vi "Visualizacion_NEW.vi"() -> ()   [LabVIEW 2022 SP3]
uses:
  4cb8985d-a683-42ab-be0b-9e8f42a2c2d0.vi
  <vilib>/Analysis/baseanly.llb/Mean (DBL).vi
  <vilib>/Modbus/master/Create Master Instance (TCP).vi
  <vilib>/Comparison/Less/Less Functor/Less Functor.lvclass
  <vilib>/Modbus/master/Modbus Master.lvclass
  <vilib>/Analysis/NI_AALBase.lvlib
panel:
  out "Temp V8":dbl(slide) scale=-40.0..100.0
  out "Temp BOB8":dbl(slide) scale=-40.0..100.0
  out "Temp BOB7":dbl(slide) scale=-40.0..100.0
  out "Temp V7":dbl(slide) scale=-40.0..100.0
  out "Temp V6":dbl(slide) scale=-40.0..100.0
  out "Temp BOB6":dbl(slide) scale=-40.0..100.0
  out "Temp BOB5":dbl(slide) scale=-40.0..100.0
  out "Temp V5":dbl(slide) scale=-40.0..100.0
  out "Temp BOB4":dbl(slide) scale=-40.0..100.0
  out "Temp V4":dbl(slide) scale=-40.0..100.0
  out "Temp V3":dbl(slide) scale=-40.0..100.0
  out "Temp BOB3":dbl(slide) scale=-40.0..100.0
  out "Temp BOB2":dbl(slide) scale=-40.0..100.0
  out "Temp V2":dbl(slide) scale=-40.0..100.0
  out "Temp V1":dbl(slide) scale=-40.0..100.0
  out "Temp BOB1":dbl(slide) scale=-40.0..100.0
  in  "Activar sim Bitron":bool
  out "MEDIA TEMPERATURAS":dbl format="%0.2f"
  out "Peltiers enable":bool
  out "Program Status":bool
  out "SP (T)":sgl
  out "Segmento_temp":u16
  in  "?":T1(tab)
  in  "?":T2(tab)
  out "TEMPERATURA MEDIA":dynamicdata(graph)
  out "ALL TOGETHER":dynamicdata(graph)
  out "VALVULA 1 Y BOBINA 1":dynamicdata(graph)
  out "VALVULA 2 Y BOBINA 2":dynamicdata(graph)
  out "VALVULA 3 Y BOBINA 3":dynamicdata(graph)
  out "VALVULA 4 Y BOBINA 4":dynamicdata(graph)
  out "VALVULA 5  Y BOBINA 5":dynamicdata(graph)
  out "VALVULA 6 Y BOBINA 6":dynamicdata(graph)
  out "VALVULA 7 Y BOBINA 7":dynamicdata(graph)
  out "VALVULA 8 Y PELTIER 8":dynamicdata(graph)
  out "Camara climatica":dynamicdata(graph)
  out "W1.16":bool
  out "W1.15":bool
  out "W1.11":bool
  out "1.10":bool
  out "W1.14":bool
  out "W1.13":bool
  out "W1.12":bool
  out "W1.1":bool
  out "W2":bool
  out "W3":bool
  out "W4":bool
  out "W1.2":bool
  out "W1.3":bool
  out "W1.6":bool
  out "W1.5":bool
  out "W1.4":bool
  out "W1.9":bool
  out "W1.8":bool
  out "W1.7":bool
  out "warnings table":T3(array[cluster]) {"Time Stamp" format="%<%.3X %x>T"}
  in  "Reset":bool
  in  "Pelt ºC/min":dbl=2.5
  in  "Cam ºC/min":dbl=2.2
  in  "Tiempo máximo de ciclo(min)":dbl=90.0
  in  "Setpoint corte frío(ºC)":dbl=-30.0
  in  "Setpoint Frío(ºC)":dbl=-40.0
  in  "Setpoint peltiers(ºC)":dbl=85.0
  in  "Tiempo estabilidad de Frío(min)":dbl=15.0
  in  "Tiempo mínimo de ciclo(min)":dbl=70.0
  in  "Setpoint calor corte rampa(ºC)":dbl=51.0
  in  "T ciclo (Bitron FSM Sim)":dbl=90.0
  in  "Setpoint calor cam":dbl=55.0
  in  "Save Parameters":bool
  out "DO H2 Lab":bool
  in  "?":T4(tab)
  out "Temp Valve 1":sgl format="%#.2g"
  out "Temp Bobina 1":sgl
  out "PWM 1(SP)":u16
  out "PWM 2(SP)":u16
  out "Temp Valve 2":sgl format="%#.2g"
  out "Temp Bobina 2":sgl
  out "PWM 3(SP)":u16
  out "Temp Valve 3":sgl format="%#.2g"
  out "Temp Bobina 3":sgl
  out "PWM 4(SP)":u16
  out "Temp Valve 4":sgl format="%#.2g"
  out "Temp Bobina 4":sgl
  out "Temp Valve 5":sgl
  out "Temp Bobina 5":sgl
  out "PWM 5(SP)":u16
  out "PWM 6(SP)":u16
  out "Temp Valve 6":sgl format="%#.2g"
  out "Temp Bobina 6":sgl
  out "PWM 7(SP)":u16
  out "Temp Valve 7":sgl format="%#.2g"
  out "Temp Bobina 7":sgl
  out "PWM 8(SP)":u16
  out "Temp Bobina 8":sgl
  out "Temp Valve 8":sgl format="%#.2g"
  in  "Guardar datos":bool=TRUE
  out "Array":dbl[][](array[numeric])
  out "Guardando en disco":bool
  out "array w/ subset deleted":dbl[][](array[numeric])
  out "Guardar Array":dbl[][](array[numeric])
  out "size(s)":i32
  out "senal_bitron":bool
  in  "Stop Control Program":bool
  out "Coils write":bool[](array[boolean])
  out "error out":errorcluster
  out "Int values":u16[](array[numeric])
  out "SGL values":sgl[](array[numeric])
  out "coil values":bool[](array[boolean])
  out "ComunicacionCRIO":bool
  out "current time":timestamp
  in  "run_program":bool
  out "Setpoint_temp_write":dbl
  out "Setpoint_hum_write":dbl
  out "Setpoint_temp_read":dbl
  out "Setpoint_hum_read":dbl
  in  "Pause_Entrar_camara":bool
  in  "Pause":bool
  in  "stop":bool
  # "Control Programa Principal"
  # "Cámara climática"
  # "ºC"
  # "ºC"
  # "%"
  # "%"
  # "Simulación señal Bitron"
  # "ºC"
  # "1            2          3           4           5          6          7          8"
  # "T Manifolds"
  # "1            2          3           4           5          6          7          8"
  # "T Bobinas"
  # "Warnings y Errores"
  # "Parametros y configuracion para la curva de ciclado"
  # "Peltier 1"
  # "ºC"
  # "ºC"
  # "Peltier 2"
  # "ºC"
  # "ºC"
  # "Peltier 3"
  # "ºC"
  # "ºC"
  # "Peltier 4"
  # "ºC"
  # "ºC"
  # "Peltier 5 (Doble)"
  # "ºC"
  # "ºC"
  # "Peltier 6 (Doble)"
  # "ºC"
  # "ºC"
  # "Peltier 7 (Doble)"
  # "ºC"
  # "ºC"
  # "Peltier 8 (Doble)"
  # "ºC"
  # "ºC"
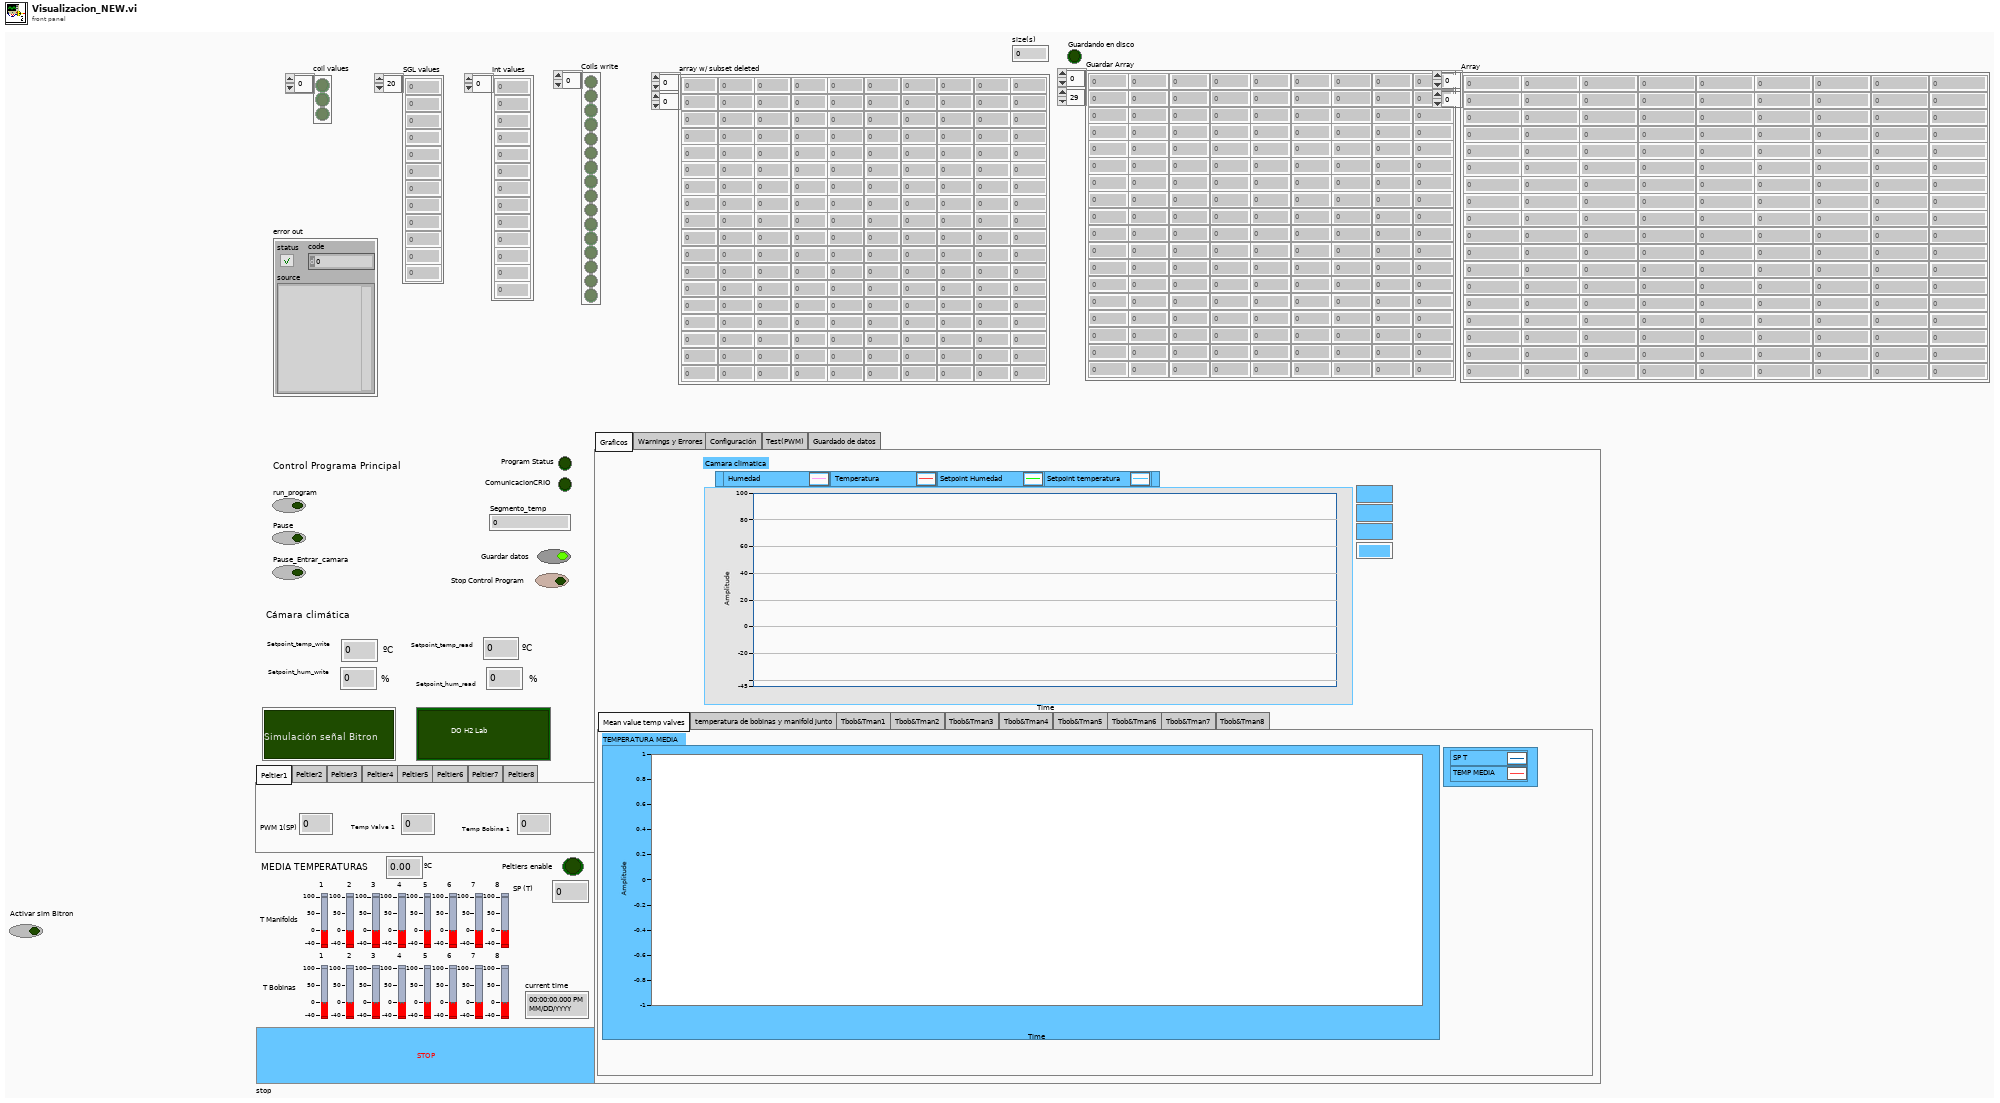
[diagram p1: front panel]
types:
  T1 = enum32{"Graficos", "Warnings y Errores", "Configuración", "Test(PWM)", "Guardado de datos"}
  T2 = enum32{"Mean value temp valves", "temperatura de bobinas y manifold junto", "Tbob&Tman1", "Tbob&Tman2", "Tbob&Tman3", "Tbob&Tman4", "Tbob&Tman5", "Tbob&Tman6", "Tbob&Tman7", "Tbob&Tman8"}
  T3 = cluster{"Time Stamp":timestamp, "Descripcion":string, "Numeric":i32}[]
  T4 = enum32{"Peltier1", "Peltier2", "Peltier3", "Peltier4", "Peltier5", "Peltier6", "Peltier7", "Peltier8"}
  T5 = enum16{"open", "open or create", "create or replace", "create", "open (read-only)"}
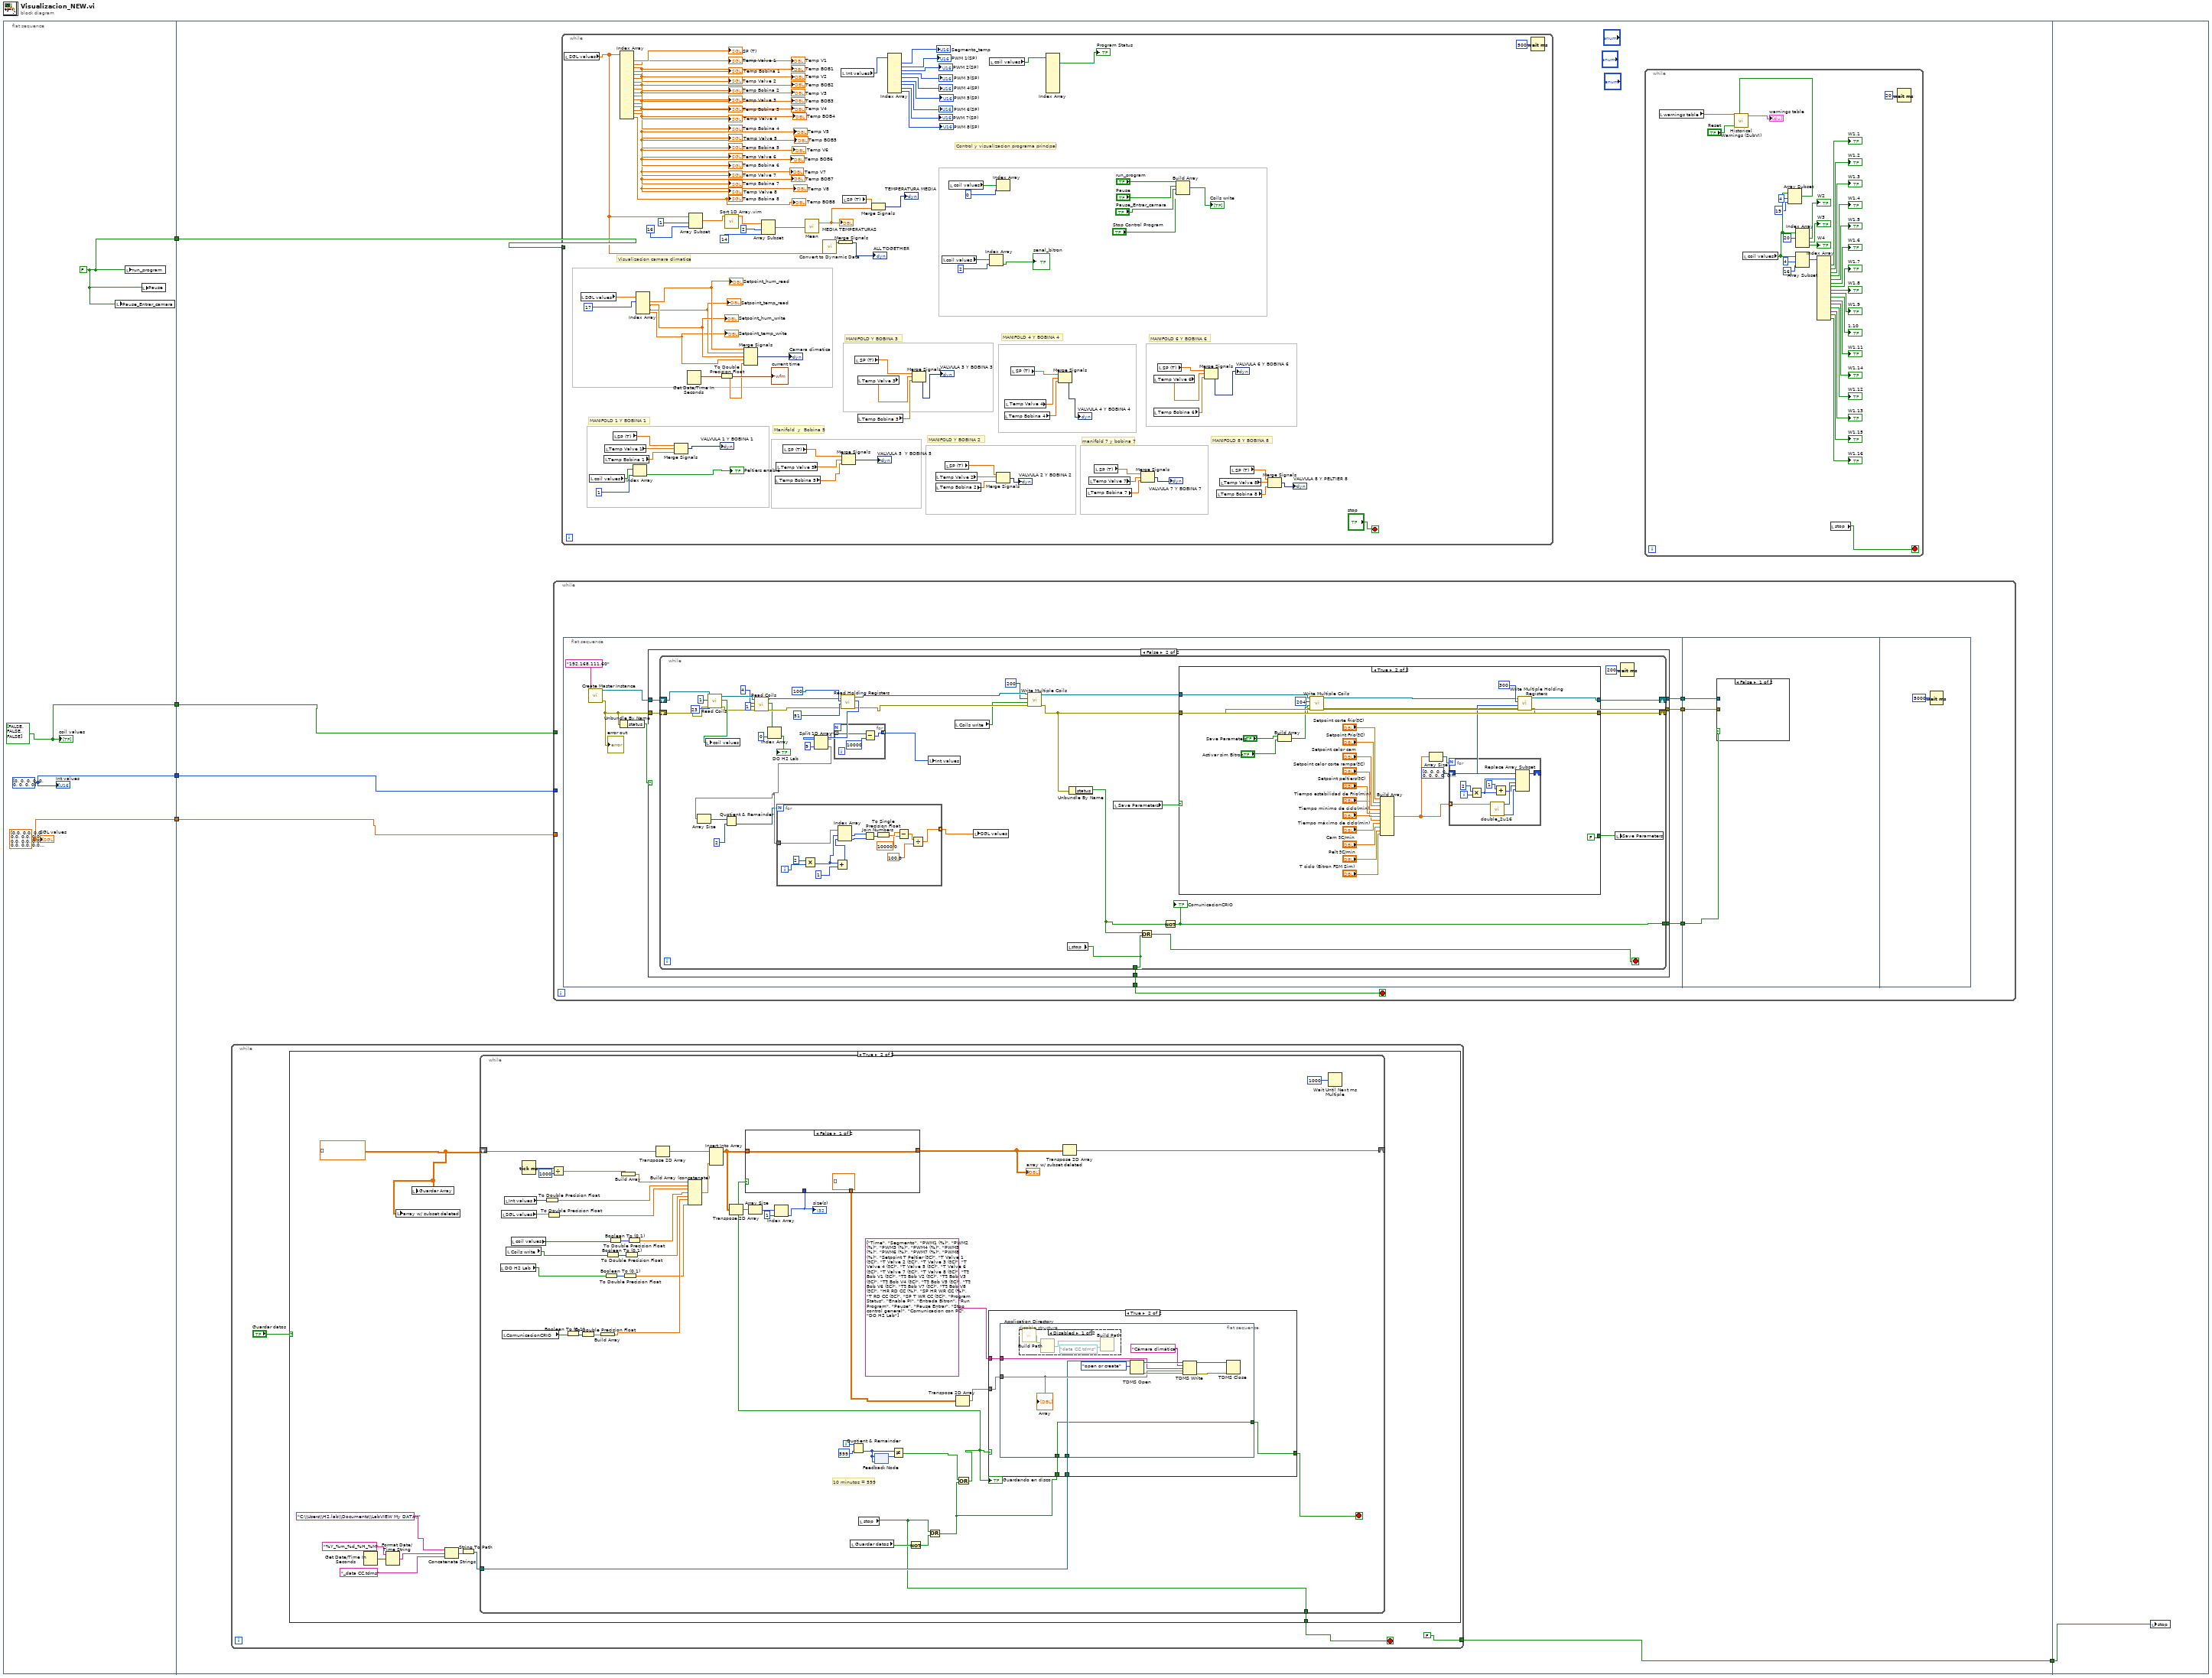
[diagram p0: block diagram]
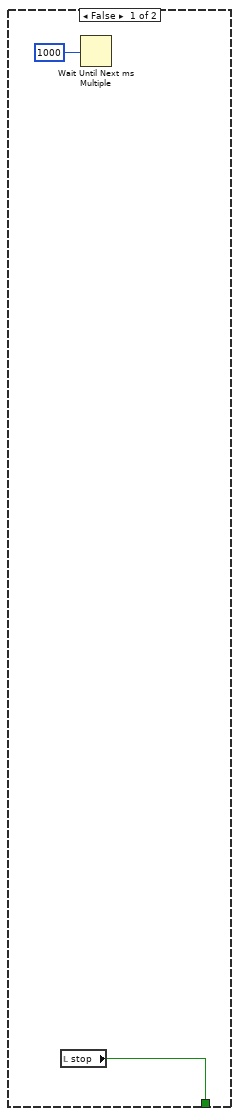
[diagram p2: hidden frame]
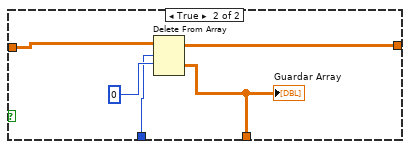
[diagram p3: hidden frame]
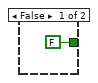
[diagram p4: hidden frame]
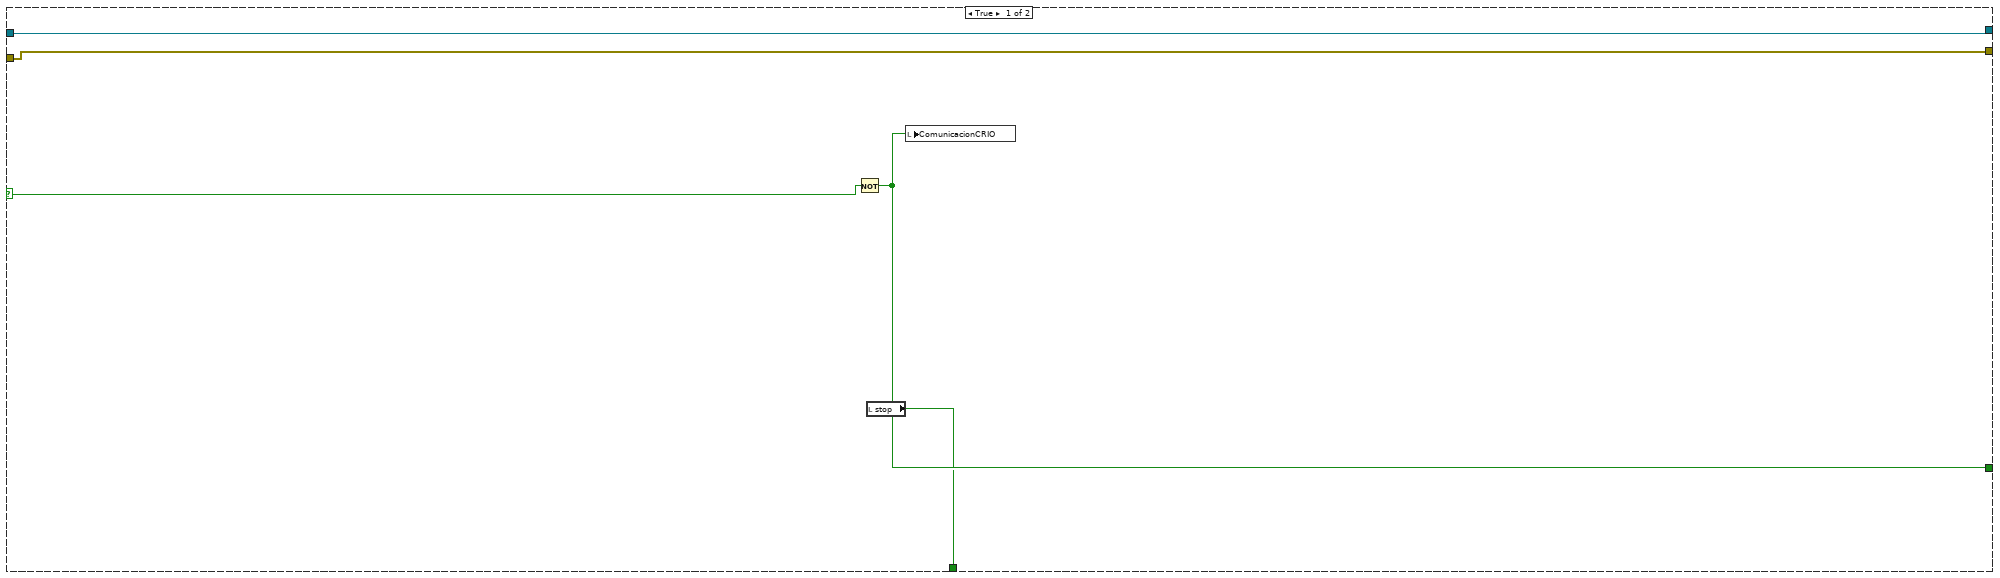
[diagram p6: hidden frame]
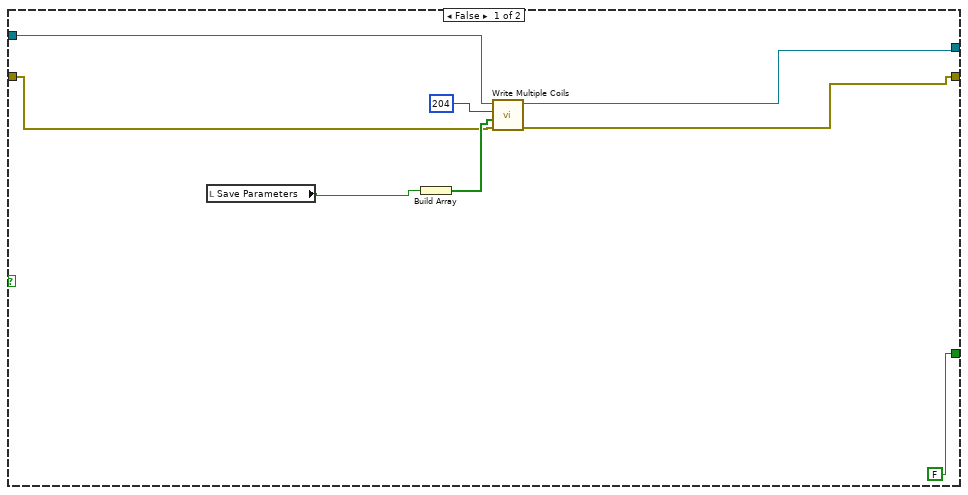
[diagram p7: hidden frame]
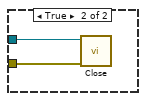
[diagram p8: hidden frame]
diagram:
  n1 = flat-sequence {
    tunnel: [w9] -> w5
    tunnel: [w8] -> w4
    tunnel: [w7] -> w3
    tunnel: [w6] -> w2
    tunnel: w5 -> [w14]
    tunnel: w4 -> [w13]
    tunnel: w3 -> [w12]
    tunnel: w2 -> [w11]
    tunnel: [w10] -> w1
    tunnel: w1 -> [w363]
    frame #0 {
      w7 = sgl[] [0.0, 0.0, 0.0, 0.0, 0.0, 0.0, 0.0, 0.0, 0.0, 0.0, 0.0, 0.0, 0.0, 0.0, 0.0, 0.0, 0.0, 0.0, 0.0, 0.0, 0.0] ("SGL values")
      w8 = u16[] [0, 0, 0, 0, 0, 0, 0, 0, 0] ("Int values")
      w6 = FALSE ("run_program")
      w9 = bool[] [FALSE, FALSE, FALSE] ("coil values")
      n2 = local write "Pause_Entrar_camara"(w6) -> ()
      n3 = local write "run_program"(w6) -> ()
      n4 = local write "Pause"(w6) -> ()
      "coil values" <- w9
      "Int values" <- w8
      "SGL values" <- w7
    }
    frame #1 {
      n5 = while {
        tunnel: [FALSE ("stop Control General")] -> w10
        stop <- w48 stop-if-true
        n6 = case shown="True" "Guardar datos" {
          tunnel: [w50 w52] -> w48
          frame False {
            n7 = local read "stop"() -> (w50:bool)
            n8 = Wait Until Next ms Multiple(millisecond multiple=u32 1000 ("milliseconds to wait")) -> ()  [unwired: 1 out]
          }
          frame True {
            w60 = dbl[][] []
            n9 = Get Date/Time In Seconds() -> (seconds since 1Jan1904=w59:timestamp)
            n10 = Format Date/Time String(time format string (%c)="%Y_%m_%d_%H_%M", seconds (now)=w59) -> (date/time string=w56:string)  [unwired: 1 in]
            n11 = local write "array w/ subset deleted"(w60) -> ()
            n12 = local write "Guardar Array"(w60) -> ()
            n13 = Concatenate Strings("C:\\Users\\H2.lab\\Documents\\LabVIEW My DATA\\" ("string"), w56, "_data CC.tdms" ("string")) -> (w57:string)
            n14 = String To Path(string=w57) -> (path=w54:path)
            n15 = while {
              shift-right: [w97] -> _
              shift-left: w60 -> [w100]
              tunnel: w54 -> [w88]
              tunnel: [w64] -> w52
              i -> [w105]
              stop <- w68 stop-if-true
              # "10 minutos = 599"
              n16 = local read "DO H2 Lab"() -> (w62:bool)
              n17 = local read "SGL values"() -> (w86:sgl[])
              n18 = local read "ComunicacionCRIO"() -> (w70:bool)
              n19 = local read "Int values"() -> (w87:u16[])
              n20 = local read "Coils write"() -> (w72:bool[])
              n21 = local read "coil values"() -> (w75:bool[])
              n22 = Tick Count (ms)() -> (millisecond timer value=w91:u32)
              n23 = To Double Precision Float(number=w87) -> (double precision float=w85:dbl[])
              n24 = To Double Precision Float(number=w86) -> (double precision float=w84:dbl[])
              n25 = Divide(x=w91, y=u32 1000) -> (x/y=w83:dbl)
              n26 = Boolean To (0,1)(Boolean=w70) -> (0, 1=w79:i16)
              n27 = To Double Precision Float(number=w79) -> (double precision float=w78:dbl)
              n28 = Build Array(w78) -> (w74:dbl[])
              n29 = Boolean To (0,1)(Boolean=w62) -> (0, 1=w63:i16)
              n30 = Boolean To (0,1)(Boolean=w72) -> (0, 1=w73:i16[])
              n31 = Boolean To (0,1)(Boolean=w75) -> (0, 1=w81:i16[])
              n32 = Build Array(w83) -> (w82:dbl[])
              n33 = To Double Precision Float(number=w63) -> (double precision float=w61:dbl)
              n34 = To Double Precision Float(number=w73) -> (double precision float=w71:dbl[])
              n35 = To Double Precision Float(number=w81) -> (double precision float=w80:dbl[])
              n36 = Transpose 2D Array(2D array=w100) -> (transposed array=w99:dbl[][])
              n37 = Build Array (concatenate)(w82, w85, w84, w80, w71, w74, w61) -> (w106:dbl[])
              n38 = Insert Into Array(array=w99, new element=w106) -> (w102:dbl[][])  [unwired: 2 in]
              n39 = Transpose 2D Array(2D array=w102) -> (transposed array=w96:dbl[][])
              n40 = Array Size(array=w96) -> (size(s)=w95:i32[])
              n41 = Index Array(array=w95, index=1) -> (element=w94:i32)
              "size(s)" <- w94
              n42 = local read "Guardar datos"() -> (w67:bool)
              n43 = Quotient & Remainder(x=w105, y=599) -> (floor(x/y)=w101:i32)  [unwired: 1 out]
              n44 = local read "stop"() -> (w64:bool)
              n45 = feedback-in #1(w101) -> ()
              n46 = feedback #1(w101) -> (w103:i32)
              n47 = Not Equal?(x=w101, y=w103) -> (x != y?=w69:bool)
              n48 = Not(x=w67) -> (.not. x?=w66:bool)
              n49 = Or(x=w64, y=w66) -> (x .or. y?=w65:bool)
              n50 = Or(x=w69, y=w65) -> (x .or. y?=w77:bool)
              "Guardando en disco" <- w77
              n51 = case shown="False" w77 {
                tunnel: w102 -> [w109 w112]
                tunnel: [w109 w114] -> w98
                tunnel: w94 -> [_ w111]
                tunnel: [dbl[][] [] w110] -> w76
                frame False {
                }
                frame True {
                  n52 = Delete From Array(array=w112, length=w111, index (row)=0) -> (deleted portion=w110:dbl[][], array with subset deleted=w114:dbl[][])  [unwired: 1 in]
                  "Guardar Array" <- w110
                }
              }
              "array w/ subset deleted" <- w98
              n53 = Transpose 2D Array(2D array=w76) -> (transposed array=w92:dbl[][])
              n54 = case shown="True" w77 {
                tunnel: string[] ["Time", "Segmento", "PWM1 (%)", "PWM2 (%)", "PWM3 (%)", "PWM4 (%)", "PWM5 (%)", "PWM6 (%)", "PWM7 (%)", "PWM8 (%)", "Setpoint T Peltier (ºC)", "T Valve 1 (ºC)", "T Valve 2 (ºC)", "T Valve 3 (ºC)", "T Valve 4 (ºC)", "T Valve 5 (ºC)", "T Valve 6 (ºC)", "T Valve 7 (ºC)", "T Valve 8 (ºC)", "Tª Bob V1 (ºC)", "Tª Bob V2 (ºC)", "Tª Bob V3 (ºC)", "Tª Bob V4 (ºC)", "Tª Bob V5 (ºC)", "Tª Bob V6 (ºC)", "Tª Bob V7 (ºC)", "Tª Bob V8 (ºC)", "HR RD CC (%)", "SP HR WR CC (%)", "T RD CC (ºC)", "SP T WR CC (ºC)", "Program Status", "Enable PI", "Entrada Bitron", "Run Program", "Pause", "Pause Entrar", "Stop control general", "Comunicacion con PC", "DO H2 Lab"] -> [_ w120]
                tunnel: w92 -> [_ w119]
                tunnel: w88 -> [_ w118]
                tunnel: w65 -> [_ w117]
                tunnel: [FALSE ("STOP ALL") w116] -> w68
                frame False {
                }
                frame True {
                  n55 = flat-sequence {
                    tunnel: w120 -> [w126]
                    tunnel: w119 -> [w123]
                    tunnel: w118 -> [w122]
                    tunnel: w117 -> [w121]
                    tunnel: [w121] -> w116
                    frame #0 {
                      n56 = disable-structure shown="Disabled" {
                        frame Disabled {
                          n57 = call <vilib>:"Application Directory.vi"() -> ("Application Directory"=w132:path)
                          n58 = Build Path(base path=w132) -> (appended path=w131:path)  [unwired: 1 in]
                          n59 = Build Path(base path=w131, name or relative path=path "data CC.tdms") -> ()  [unwired: 1 out]
                        }
                        frame Enabled {
                        }
                      }
                      n60 = TDMS Open(10:T5."open or create" ("operation (0:open)"), 11:w122) -> (0:w128:errorcluster, 3:w129:refnum<k34>)  [unwired: 5 in]
                      n61 = TDMS Write(0:w129, 5:"Cámara climática" ("group name in (Untitled)"), 7:w126, 9:w123, 11:w128) -> (4:w125:refnum<k34>, 15:w124:errorcluster)  [unwired: 1 in, 2 out]
                      n62 = TDMS Close(8:w124, 11:w125) -> ()  [unwired: 2 out]
                      "Array" <- w123
                    }
                  }
                }
              }
              n63 = Transpose 2D Array(2D array=w98) -> (transposed array=w97:dbl[][])
              n64 = Wait Until Next ms Multiple(millisecond multiple=u32 1000 ("milliseconds to wait")) -> ()  [unwired: 1 out]
            }
          }
        }
      }
      n65 = while {
        tunnel: w14 -> [_]
        tunnel: w13 -> [_]
        tunnel: w12 -> [_]
        stop <- w134 stop-if-true
        n66 = flat-sequence {
          tunnel: [w143] -> w137
          tunnel: [w142] -> w136
          tunnel: [w141] -> w135
          tunnel: [w140] -> w134
          tunnel: w137 -> [w261]
          tunnel: w136 -> [w260]
          tunnel: w135 -> [w259]
          frame #0 {
            n67 = call-poly <vilib>:"Create Master Instance.vi"("address"="192.168.111.60") -> ("error out"=w139:errorcluster, "TCP master instance"=w144:refnum<class "Modbus Master.lvclass">)  [unwired: 9 in]
            "error out" <- w139
            n68 = Unbundle By Name(w139) -> ("status"=w138:bool)
            n69 = case shown="False" w138 {
              selector: w138 -> [w147 _]
              tunnel: w144 -> [w150 w156]
              tunnel: [w148 w155] -> w143
              tunnel: [w150 w154] -> w142
              tunnel: [w149 w153] -> w141
              tunnel: [w146 w152] -> w140
              tunnel: w139 -> [w149 w151]
              frame True {
                n70 = Not(x=w147) -> (.not. x?=w148:bool)
                n71 = local read "stop"() -> (w146:bool)
                n72 = local write "ComunicacionCRIO"(w148) -> ()
              }
              frame False {
                n73 = while {
                  shift-right: [w158] -> w154
                  shift-left: w156 -> [w185]
                  shift-right: [w157] -> w153
                  shift-left: w151 -> [w184]
                  tunnel: [w181] -> w155
                  tunnel: [w179] -> w152
                  stop <- w183 stop-if-true
                  n74 = call-dynamic "Read Coils.vi"("error in (no error)"=w184, "number of coils"=u16 23, "starting address"=u16 1, "Modbus master in"=w185) -> ("error out"=w170:errorcluster, "coil values"=w174:bool[], "Modbus master out"=w171:refnum<class "Modbus Master.lvclass">)  [unwired: 5 in]
                  n75 = local write "coil values"(w174) -> ()
                  n76 = call-dynamic "Read Coils.vi"("error in (no error)"=w170, "number of coils"=u16 1, "starting address"=u16 4, "Modbus master in"=w171) -> ("error out"=w168:errorcluster, "coil values"=w165:bool[], "Modbus master out"=w169:refnum<class "Modbus Master.lvclass">)  [unwired: 5 in]
                  n77 = Index Array(array=w165, index=0) -> (element=→"DO H2 Lab":bool)
                  n78 = call-dynamic "Read Holding Registers.vi"("error in (no error)"=w168, "number of holding registers"=u16 51, "starting address"=u16 100, "Modbus master in"=w169) -> ("error out"=w177:errorcluster, "register values"=w187:u16[], "Modbus master out"=w178:refnum<class "Modbus Master.lvclass">)  [unwired: 5 in]
                  n79 = Split 1D Array(array=w187, index=9) -> (first subarray=w186:u16[], second subarray=w191:u16[])
                  n80 = Array Size(array=w191) -> (size(s)=w190:i32)
                  n81 = Quotient & Remainder(x=w190, y=2) -> (floor(x/y)=w188:i32)  [unwired: 1 out]
                  n82 = for {
                    N: w188 -> [_]
                    tunnel: w191 -> [w251]
                    tunnel: [w248] -> w172 mode=indexing
                    i -> [w258]
                    n83 = Multiply(x=2, y=w258) -> (x*y=w256:i32)
                    n84 = Add(x=w256, y=1) -> (x+y=w254:i32)
                    n85 = Index Array(array=w251, index #1=w256, index #2=w254) -> (element #1=w253:u16, element #2=w252:u16)
                    n86 = Join Numbers(hi=w253, lo=w252) -> ((hi.lo)=w250:u32)
                    n87 = To Single Precision Float(number=w250) -> (single precision float=w247:sgl)
                    n88 = Subtract(x=w247, y=sgl 10000.0) -> (x-y=w245:sgl)
                    n89 = Divide(x=w245, y=sgl 100.0) -> (x/y=w248:sgl)
                  }
                  n90 = for {
                    tunnel: w186 -> [w244] mode=indexing
                    tunnel: [w242] -> w173 mode=indexing
                    n91 = Subtract(x=w244, y=u16 10000) -> (x-y=w242:u16)
                  }
                  n92 = local write "Int values"(w173) -> ()
                  n93 = local read "Coils write"() -> (w175:bool[])
                  n94 = local write "SGL values"(w172) -> ()
                  n95 = call-dynamic "Write Multiple Coils.vi"("error in (no error)"=w177, "coil values"=w175, "starting address"=u16 200, "Modbus master in"=w178) -> ("error out"=w159:errorcluster, "Modbus master out"=w160:refnum<class "Modbus Master.lvclass">)  [unwired: 6 in]
                  n96 = local read "stop"() -> (w179:bool)
                  n97 = Unbundle By Name(w159) -> ("status"=w182:bool)
                  n98 = local read "Save Parameters"() -> (w162:bool)
                  n99 = Or(x=w182, y=w179) -> (x .or. y?=w183:bool)
                  n100 = Not(x=w182) -> (.not. x?=w181:bool)
                  "ComunicacionCRIO" <- w181
                  n101 = case shown="True" w162 {
                    tunnel: [FALSE ("Save Parameters") FALSE ("Save Parameters")] -> w161
                    tunnel: w160 -> [w200 w208]
                    tunnel: w159 -> [w199 w207]
                    tunnel: [w198 w206] -> w158
                    tunnel: [w197 w205] -> w157
                    frame False {
                      n102 = local read "Save Parameters"() -> (w201:bool)
                      n103 = Build Array(w201) -> (w203:bool[])
                      n104 = call-dynamic "Write Multiple Coils.vi"("error in (no error)"=w199, "coil values"=w203, "starting address"=u16 204, "Modbus master in"=w200) -> ("error out"=w197:errorcluster, "Modbus master out"=w198:refnum<class "Modbus Master.lvclass">)  [unwired: 6 in]
                    }
                    frame True {
                      n105 = Build Array("Save Parameters", "Activar sim Bitron") -> (w212:bool[])
                      n106 = call-dynamic "Write Multiple Coils.vi"("error in (no error)"=w207, "coil values"=w212, "starting address"=u16 204, "Modbus master in"=w208) -> ("error out"=w211:errorcluster, "Modbus master out"=w210:refnum<class "Modbus Master.lvclass">)  [unwired: 6 in]
                      n107 = Build Array("Setpoint corte frío(ºC)", "Setpoint Frío(ºC)", "Setpoint calor cam", "Setpoint calor corte rampa(ºC)", "Setpoint peltiers(ºC)", "Tiempo estabilidad de Frío(min)", "Tiempo mínimo de ciclo(min)", "Tiempo máximo de ciclo(min)", "Cam ºC/min", "Pelt ºC/min", "T ciclo (Bitron FSM Sim)") -> (w219:dbl[])
                      n108 = Array Size(array=w219) -> (size(s)=w218:i32)
                      n109 = for {
                        N: w218 -> [_]
                        shift-right: [w233] -> w216
                        shift-left: u16[] [0, 0, 0, 0, 0, 0, 0, 0, 0, 0, 0, 0, 0, 0, 0, 0, 0, 0, 0, 0, 0, 0] -> [w234]
                        tunnel: w219 -> [w232] mode=indexing
                        i -> [w241]
                        n110 = Multiply(x=2, y=w241) -> (x*y=w237:i32)
                        n111 = call "double_2u16.vi"("Entrada"=w232) -> ("Salida 2"=w238:u16, "Salida 1"=w239:u16)  [unwired: 9 in]
                        n112 = Add(x=1, y=w237) -> (x+y=w235:i32)
                        n113 = Replace Array Subset(array=w234, new element #1=w239, index #1=w237, new element #2=w238, index #2=w235) -> (w233:u16[])
                      }
                      n114 = call-dynamic "Write Multiple Holding Registers.vi"("error in (no error)"=w211, "holding register values"=w216, "starting address"=u16 300, "Modbus master in"=w210) -> ("error out"=w205:errorcluster, "Modbus master out"=w206:refnum<class "Modbus Master.lvclass">)  [unwired: 6 in]
                    }
                  }
                  n115 = local write "Save Parameters"(w161) -> ()
                  n116 = Wait (ms)(milliseconds to wait=u32 200) -> ()  [unwired: 1 out]
                }
              }
            }
          }
          frame #1 {
            n117 = case shown="False" w261 {
              tunnel: w260 -> [_ w263]
              tunnel: w259 -> [_ w262]
              frame False {
              }
              frame True {
                n118 = call-dynamic "Close.vi"("error in (no error)"=w262, "Modbus master in"=w263) -> ()  [unwired: 9 in, 1 out]
              }
            }
          }
          frame #2 {
            n119 = Wait (ms)(milliseconds to wait=u32 5000) -> ()  [unwired: 1 out]
          }
        }
      }
      n120 = while {
        tunnel: w11 -> [_]
        stop <- "stop" stop-if-true
        # "MANIFOLD 8 Y BOBINA 8"
        # "manifold 7 y bobina 7"
        # "MANIFOLD 6 Y BOBINA 6"
        # "MANIFOLD 4 Y BOBINA 4"
        # "MANIFOLD Y BOBINA 3"
        # "MANIFOLD Y BOBINA 2"
        # "Manifold  y  Bobina 5"
        # "MANIFOLD 1 Y BOBINA 1"
        # "Visualizacion camara climatica"
        # "Control y visualizacion programa principal"
        n121 = local read "SGL values"() -> (w283:sgl[])
        n122 = local read "SGL values"() -> (w357:sgl[])
        n123 = local read "coil values"() -> (w351:bool[])
        n124 = local read "Temp Bobina 1"() -> (w334:sgl)
        n125 = local read "Temp Valve 1"() -> (w335:sgl)
        n126 = local read "SP (T)"() -> (w336:sgl)
        n127 = Index Array(array=w283) -> (element #1=→"SP (T)":sgl, element #2=→"Temp Valve 1" →"Temp V1":sgl, element #3=→"Temp Bobina 1" →"Temp BOB1":sgl, element #4=→"Temp Valve 2" →"Temp V2":sgl, element #5=→"Temp Bobina 2" →"Temp BOB2":sgl, element #6=→"Temp Valve 3" →"Temp V3":sgl, element #7=→"Temp Bobina 3" →"Temp BOB3":sgl, element #8=→"Temp Valve 4" →"Temp V4":sgl, element #9=→"Temp Bobina 4" →"Temp BOB4":sgl, element #10=→"Temp Valve 5" →"Temp V5":sgl, element #11=→"Temp Bobina 5" →"Temp BOB5":sgl, element #12=→"Temp Valve 6" →"Temp V6":sgl, element #13=→"Temp Bobina 6" →"Temp BOB6":sgl, element #14=→"Temp Valve 7" →"Temp V7":sgl, element #15=→"Temp Bobina 7" →"Temp BOB7":sgl, element #16=→"Temp Valve 8" →"Temp V8":sgl, element #17=→"Temp Bobina 8" →"Temp BOB8":sgl)  [unwired: 17 in]
        n128 = Index Array(array=w351, index=1) -> (element=→"Peltiers enable":bool)
        n129 = Index Array(array=w357, index #1=17 ("index")) -> (element #1=w355:sgl, element #2=w354:sgl, element #3=w353:sgl, element #4=w352:sgl)  [unwired: 3 in]
        "Setpoint_hum_read" <- w355
        "Setpoint_temp_read" <- w353
        "Setpoint_hum_write" <- w354
        "Setpoint_temp_write" <- w352
        n130 = Merge Signals(w336, w335, w334) -> (→"VALVULA 1 Y BOBINA 1":dynamicdata)
        n131 = Get Date/Time In Seconds() -> (seconds since 1Jan1904=w360:timestamp)
        "current time" <- w360
        n132 = Array Subset(array=w283, index=1, length=16) -> (w292:sgl[])
        n133 = To Double Precision Float(number=w360) -> (double precision float=w359:dbl)
        n134 = call "Sort 1D Array.vim"("unsorted array"=w292) -> ("sorted array"=w291:sgl[])  [unwired: 10 in]
        n135 = Merge Signals(w355, w353, w354, w352, w359) -> (→"Camara climatica":dynamicdata)
        n136 = Array Subset(array=w291, index=2, length=14) -> (w288:sgl[])
        n137 = local read "Temp Bobina 5"() -> (w319:sgl)
        n138 = local read "Temp Valve 5"() -> (w320:sgl)
        n139 = local read "SP (T)"() -> (w321:sgl)
        n140 = call-poly <vilib>:"Mean.vi"("X"=w288) -> ("mean"=w286:dbl)  [unwired: 1 out]
        "MEDIA TEMPERATURAS" <- w286
        n141 = call "Convert to Dynamic Data"("Array"=w283) -> ("Dynamic Data Type"=w282:dynamicdata)  [unwired: 3 in]
        n142 = Merge Signals(w282) -> (→"ALL TOGETHER":dynamicdata)
        n143 = local read "Int values"() -> (w333:u16[])
        n144 = Merge Signals(w321, w320, w319) -> (→"VALVULA 5  Y BOBINA 5":dynamicdata)
        n145 = local read "SP (T)"() -> (w287:sgl)
        n146 = local read "SP (T)"() -> (w315:sgl)
        n147 = local read "Temp Valve 3"() -> (w314:sgl)
        n148 = local read "Temp Bobina 3"() -> (w313:sgl)
        n149 = Merge Signals(w287, w286) -> (→"TEMPERATURA MEDIA":dynamicdata)
        n150 = Index Array(array=w333) -> (element #1=→"Segmento_temp":u16, element #2=→"PWM 1(SP)":u16, element #3=→"PWM 2(SP)":u16, element #4=→"PWM 3(SP)":u16, element #5=→"PWM 4(SP)":u16, element #6=→"PWM 5(SP)":u16, element #7=→"PWM 6(SP)":u16, element #8=→"PWM 7(SP)":u16, element #9=→"PWM 8(SP)":u16)  [unwired: 9 in]
        n151 = Merge Signals(w315, w314, w313) -> (→"VALVULA 3 Y BOBINA 3":dynamicdata)
        n152 = local read "Temp Valve 2"() -> (w308:sgl)
        n153 = local read "Temp Bobina 2"() -> (w307:sgl)
        n154 = local read "coil values"() -> (w341:bool[])
        n155 = local read "SP (T)"() -> (w317:sgl)
        n156 = local read "coil values"() -> (w348:bool[])
        n157 = Index Array(array=w341, index=2) -> (element=→"senal_bitron":bool)
        n158 = local read "coil values"() -> (w323:bool[])
        n159 = Index Array(array=w348, index=0) -> ()  [unwired: 1 out]
        n160 = Merge Signals(w317, w308, w307) -> (→"VALVULA 2 Y BOBINA 2":dynamicdata)
        n161 = local read "Temp Bobina 4"() -> (w309:sgl)
        n162 = local read "Temp Valve 4"() -> (w310:sgl)
        n163 = local read "SP (T)"() -> (w311:sgl)
        n164 = Index Array(array=w323) -> (element #1=→"Program Status":bool)  [unwired: 9 in, 8 out]
        n165 = Merge Signals(w311, w310, w309) -> (→"VALVULA 4 Y BOBINA 4":dynamicdata)
        n166 = local read "Temp Bobina 7"() -> (w300:sgl)
        n167 = local read "Temp Valve 7"() -> (w301:sgl)
        n168 = local read "SP (T)"() -> (w302:sgl)
        n169 = Merge Signals(w302, w301, w300) -> (→"VALVULA 7 Y BOBINA 7":dynamicdata)
        n170 = local read "Temp Valve 6"() -> (w305:sgl)
        n171 = local read "Temp Bobina 6"() -> (w306:sgl)
        n172 = local read "SP (T)"() -> (w304:sgl)
        n173 = Build Array("run_program", "Pause", "Pause_Entrar_camara", "Stop Control Program") -> (→"Coils write":bool[])
        n174 = Merge Signals(w304, w305, w306) -> (→"VALVULA 6 Y BOBINA 6":dynamicdata)
        n175 = local read "Temp Bobina 8"() -> (w295:sgl)
        n176 = local read "Temp Valve 8"() -> (w296:sgl)
        n177 = local read "SP (T)"() -> (w297:sgl)
        n178 = Merge Signals(w297, w296, w295) -> (→"VALVULA 8 Y PELTIER 8":dynamicdata)
        n179 = Wait (ms)(milliseconds to wait=u32 500) -> ()  [unwired: 1 out]
      }
      n180 = while {
        stop <- w16 stop-if-true
        n181 = local read "warnings table"() -> (w19:T3)
        n182 = local read "coil values"() -> (w45:bool[])
        n183 = Array Subset(array=w45, index=4, length=19) -> (w46:bool[])
        n184 = call "Historical Warnings (SubVI).vi"("Warnings bool array"=w46, "in"="Reset", "warnings table in"=w19) -> ("Warnings table out"=→"warnings table":T3)  [unwired: 8 in]
        n185 = Index Array(array=w45, index #1=20 ("index")) -> (element #1=→"W2":bool, element #2=→"W3":bool, element #3=→"W4":bool)  [unwired: 2 in]
        n186 = Array Subset(array=w45, index=4, length=16) -> (w28:bool[])
        n187 = Index Array(array=w28) -> (element #1=→"W1.1":bool, element #2=→"W1.2":bool, element #3=→"W1.3":bool, element #4=→"W1.4":bool, element #5=→"W1.5":bool, element #6=→"W1.6":bool, element #7=→"W1.7":bool, element #8=→"W1.8":bool, element #9=→"W1.9":bool, element #10=→"1.10":bool, element #11=→"W1.11":bool, element #12=→"W1.14":bool, element #13=→"W1.12":bool, element #14=→"W1.13":bool, element #15=→"W1.15":bool, element #16=→"W1.16":bool)  [unwired: 16 in]
        n188 = local read "stop"() -> (w16:bool)
        n189 = Wait (ms)(milliseconds to wait=u32 20) -> ()  [unwired: 1 out]
      }
    }
    frame #2 {
      n190 = local write "stop"(w363) -> ()
    }
  }
